vi "单个写入.vi"(8 "Error in":errorcluster caption="Error in (no error)", 9 "value":u16, 10 "address":u16, 11 "Slave ID":u8=10) -> (0 "error out":errorcluster)   [LabVIEW 2016, in "质控单元.lvlib"]
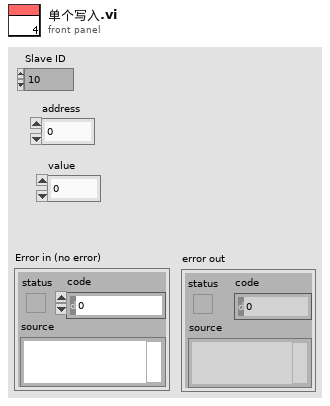
[diagram p1: front panel]
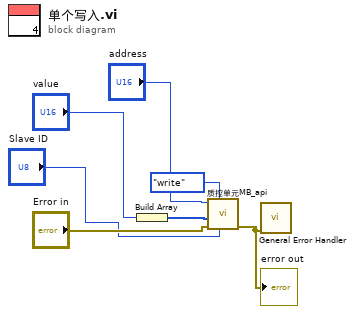
[diagram p0: block diagram]
diagram:
  n1 = Build Array("value") -> (w3:u16[])
  n2 = call "质控单元MB_api.vi"("Slave ID"="Slave ID", "STEP"=enum16{"open", "read", "write", "close"}."write", "Error in"="Error in", "values"=w3, "starting address"="address") -> ("error out"=w5:errorcluster)  [unwired: 3 in, 3 out]
  "error out" <- w5
  n3 = call <vilib>:"General Error Handler.vi"("error in (no error)"=w5) -> ()  [unwired: 10 in, 5 out]
